vi "Create Measurement Service.vi"(7 "project ref":refnum<vi>, 8 "error in (no error)":errorcluster, 10 "measurement plug-in description":string, 11 "measurement plug-in name":string) -> (0 "error out":errorcluster)   [LabVIEW 2021, in "MeasurementService Editor.lvlib"]
uses:
  _Editor/MeasurementService Editor.lvlib
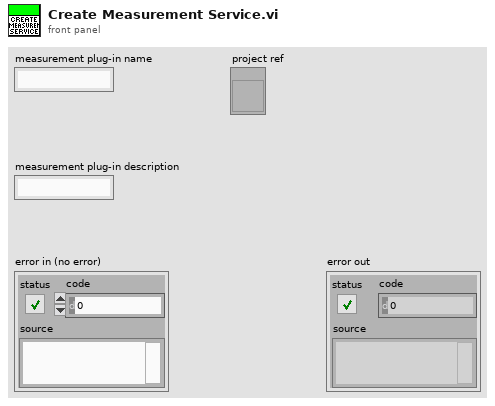
[diagram p1: front panel]
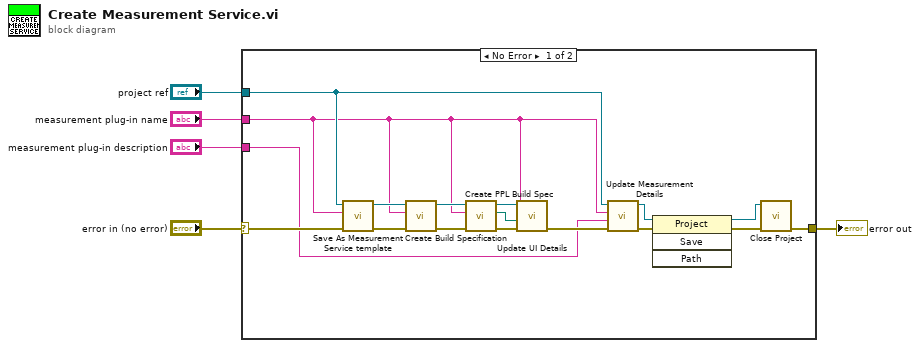
[diagram p0: block diagram]
diagram:
  n1 = case shown="No Error" "error in (no error)" {
    selector: "error in (no error)" -> [w22 w23]
    tunnel: [w21 w23] -> w4
    tunnel: "project ref" -> [w8 _]
    tunnel: "measurement plug-in name" -> [w7 _]
    tunnel: "measurement plug-in description" -> [w6 _]
    frame No Error {
      n2 = call "Save As Measurement Service template.vi"("error in"=w22, "measurement service name"=w7, "project ref"=w8) -> ("error out"=w15:errorcluster, "project ref out"=w18:refnum<vi>)  [unwired: 7 in]
      n3 = call "Create Build Specification.vi"("error in"=w15, "measurement service name"=w7, "project ref"=w18) -> ("error out"=w16:errorcluster, "project ref out"=w17:refnum<vi>)  [unwired: 7 in]
      n4 = call "Create PPL Build Spec.vi"("error in (no error)"=w16, "measurement plug-in name"=w7, "project refnum"=w17) -> ("error out"=w13:errorcluster, "measurement UI built path"=w12:path, "project ref out"=w14:refnum<vi>)  [unwired: 6 in]
      n5 = call "Update UI Details.vi"("error in"=w13, "UI path"=w12, "measurement service name"=w7, "project ref"=w14) -> ("error out"=w11:errorcluster)  [unwired: 6 in, 1 out]
      n6 = call "Update Measurement Details.vi"("error in"=w11, "measurement service description"=w6, "measurement service name"=w7, "project ref"=w8) -> ("error out"=w20:errorcluster, "project ref out"=w9:refnum<vi>)  [unwired: 6 in]
      n7 = invoke class="Project" method="Save"(reference=w9, error in=w20) -> (reference out=w10:refnum<vi>, error out=w19:errorcluster)  [unwired: 2 in, 2 out]
      n8 = call "Close Project.vi"("error in"=w19, "project ref"=w10) -> ("error out"=w21:errorcluster)  [unwired: 9 in]
    }
    frame Error {
    }
  }
  "error out" <- w4
